vi "DestroyEvents.vi"(8 "error in (no error)":errorcluster, 11 "Events":T1) -> (0 "error out":errorcluster)   [LabVIEW 2022 SP3, in "Gui.lvlib" / "Gui.lvclass"]
uses:
  Gui.lvclass
  _Events.ctl
  Gui.lvclass/Gui.ctl
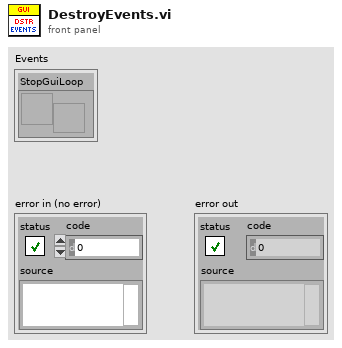
[diagram p1: front panel]
types:
  T1 = typedef "Gui.lvlib/Gui.lvclass/_Events.ctl" = cluster{"StopGuiLoop":refnum<user-event>}
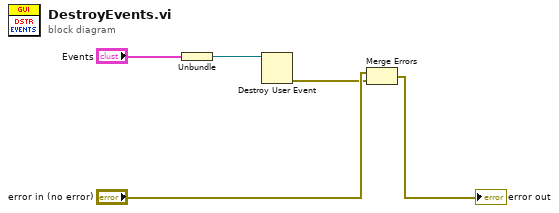
[diagram p0: block diagram]
diagram:
  n1 = Unbundle("Events") -> ("StopGuiLoop"=w4:refnum<user-event>)
  n2 = Destroy User Event(user event=w4) -> (error out=w1:errorcluster)  [unwired: 1 in]
  n3 = Merge Errors("error in (no error)", w1) -> (→"error out":errorcluster)
